vi "BuildInterface.vi"(6 "ProjectPath":path, 8 "error in (no error)":errorcluster, 9 "Application":refnum<vi>, 11 "Interface in":refnum<class "Interface.lvclass">) -> (0 "error out":errorcluster, 3 "Interface out":refnum<class "Interface.lvclass">)   [LabVIEW 2020, in "Mermaid.lvlib" / "Interface.lvclass"]
uses:
  Interface.lvclass
  Interface.lvclass/Interface.ctl
  _Class/Class.lvclass
  _CreateInterface/CreateInterface.lvclass
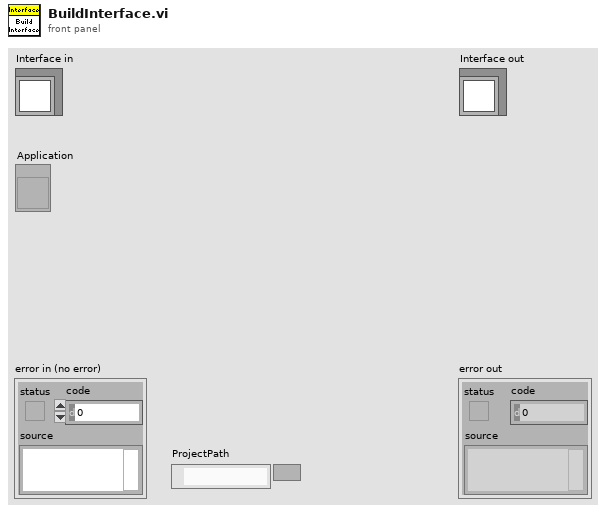
[diagram p1: front panel]
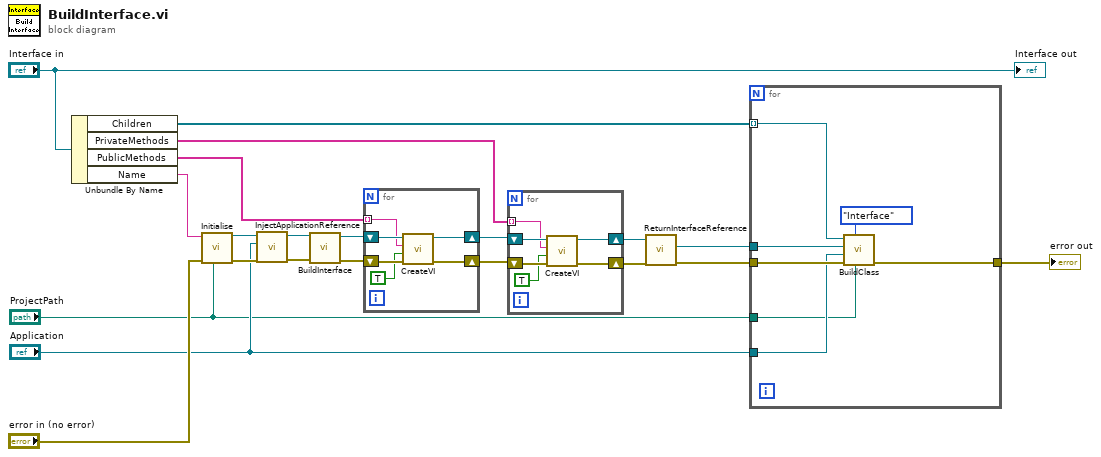
[diagram p0: block diagram]
diagram:
  n1 = Unbundle By Name("Interface in") -> ("Children"=w4:refnum<class "Class.lvclass">[], "PrivateMethods"=w9:string[], "PublicMethods"=w12:string[], "Name"=w18:string)
  n2 = call "Initialise.vi"("ProjectPath"="ProjectPath", "error in (no error)"="error in (no error)", "Interface Name"=w18) -> ("error out"=w16:errorcluster, "CreateInterface out"=w20:refnum<class "CreateInterface.lvclass">)  [unwired: 7 in]
  n3 = call "InjectApplicationReference.vi"("error in (no error)"=w16, "Application"="Application", "CreateInterface in"=w20) -> ("error out"=w15:errorcluster, "CreateInterface out"=w19:refnum<class "CreateInterface.lvclass">)  [unwired: 7 in]
  n4 = call "BuildInterface.vi"("error in (no error)"=w15, "CreateInterface in"=w19) -> ("error out"=w14:errorcluster, "CreateInterface out"=w13:refnum<class "CreateInterface.lvclass">)  [unwired: 8 in]
  n5 = for {
    tunnel: w12 -> [w26] mode=indexing
    shift-right: [w23] -> w11
    shift-left: w13 -> [w27]
    shift-right: [w22] -> w10
    shift-left: w14 -> [w25]
    n6 = call "CreateVI.vi"("error in (no error)"=w25, "Dynamic Dispatch (T)"=TRUE, "Name"=w26, "CreateInterface in"=w27) -> ("error out"=w22:errorcluster, "CreateInterface out"=w23:refnum<class "CreateInterface.lvclass">)  [unwired: 6 in]
  }
  n7 = for {
    tunnel: w9 -> [w32] mode=indexing
    shift-right: [w29] -> w7
    shift-left: w11 -> [w33]
    shift-right: [w28] -> w8
    shift-left: w10 -> [w31]
    n8 = call "CreateVI.vi"("error in (no error)"=w31, "Dynamic Dispatch (T)"=TRUE, "Name"=w32, "CreateInterface in"=w33) -> ("error out"=w28:errorcluster, "CreateInterface out"=w29:refnum<class "CreateInterface.lvclass">)  [unwired: 6 in]
  }
  n9 = call "ReturnInterfaceReference.vi"("error in (no error)"=w8, "CreateInterface in"=w7) -> ("error out"=w6:errorcluster, "IntRef"=w5:refnum<vi>)  [unwired: 7 in, 1 out]
  n10 = for {
    tunnel: w6 -> [w39]
    tunnel: w5 -> [w37]
    tunnel: "Application" -> [w36]
    tunnel: w4 -> [w40] mode=indexing
    tunnel: [w35] -> w3
    tunnel: "ProjectPath" -> [w34]
    n11 = call-dynamic "BuildClass.vi"("ProjectPath"=w34, "Parent"=enum16{"None", "Interface", "Class"}."Interface", "error in (no error)"=w39, "Application"=w36, "ParentRef"=w37, "Class in"=w40) -> ("error out"=w35:errorcluster)  [unwired: 4 in, 1 out]
  }
  "error out" <- w3
  "Interface out" <- "Interface in"
